vi "Pressure_control_subVI _newturbo.vi"(7 "Run Sequence":bool, 8 "user sequence, present (s) in, current step in, seq time in":T6, 9 "pressure parameters in":T3={"valve % open"=100.0, "Desired pressure"=0.0, "set Vapor sccm"=0.0, "set Gas sccm"=0.0, "Valve mode"=enum."% Open", "Pressure Mode"=enum."Abs. pressure", "analyte partial pressure"=100.0} caption="Set pressure parameters" {"analyte partial pressure" min=0.0 max=100.0 step=5.0; "set Gas sccm" min=0 max=200 step=5; "set Vapor sccm" min=0 max=200 step=5; "Desired pressure" min=0.0 max=760.0 step=5.0; "valve % open" min=0.0 max=100.0 step=5.0 format="%#_2f"}, 11 "pressure control on?/daq IDs/errors":T2) -> (0 "current step # out, shift register time out, seq button on?":T5, 1 "sequence over? USE THIS TO REINITIALIZE RUN SEQUENCE BUTTON SO PROGRAM ENDS":bool, 2 "save press/RH/gasflow/vaporflow - read valve position/pressure/vaporflow/gasflow":T4, 3 "pressure control on?/daq IDs/errors out":T1, 4 "sequence end date/time string":string, 5 "pressure_setpoint":string)   [LabVIEW 2014]
uses:
  <vilib>/DAQmx/read.llb/DAQmx Read (Analog 1D DBL NChan 1Samp).vi
  <vilib>/DAQmx/write.llb/DAQmx Write (Analog 1D DBL NChan 1Samp).vi
panel:
  # "100%"
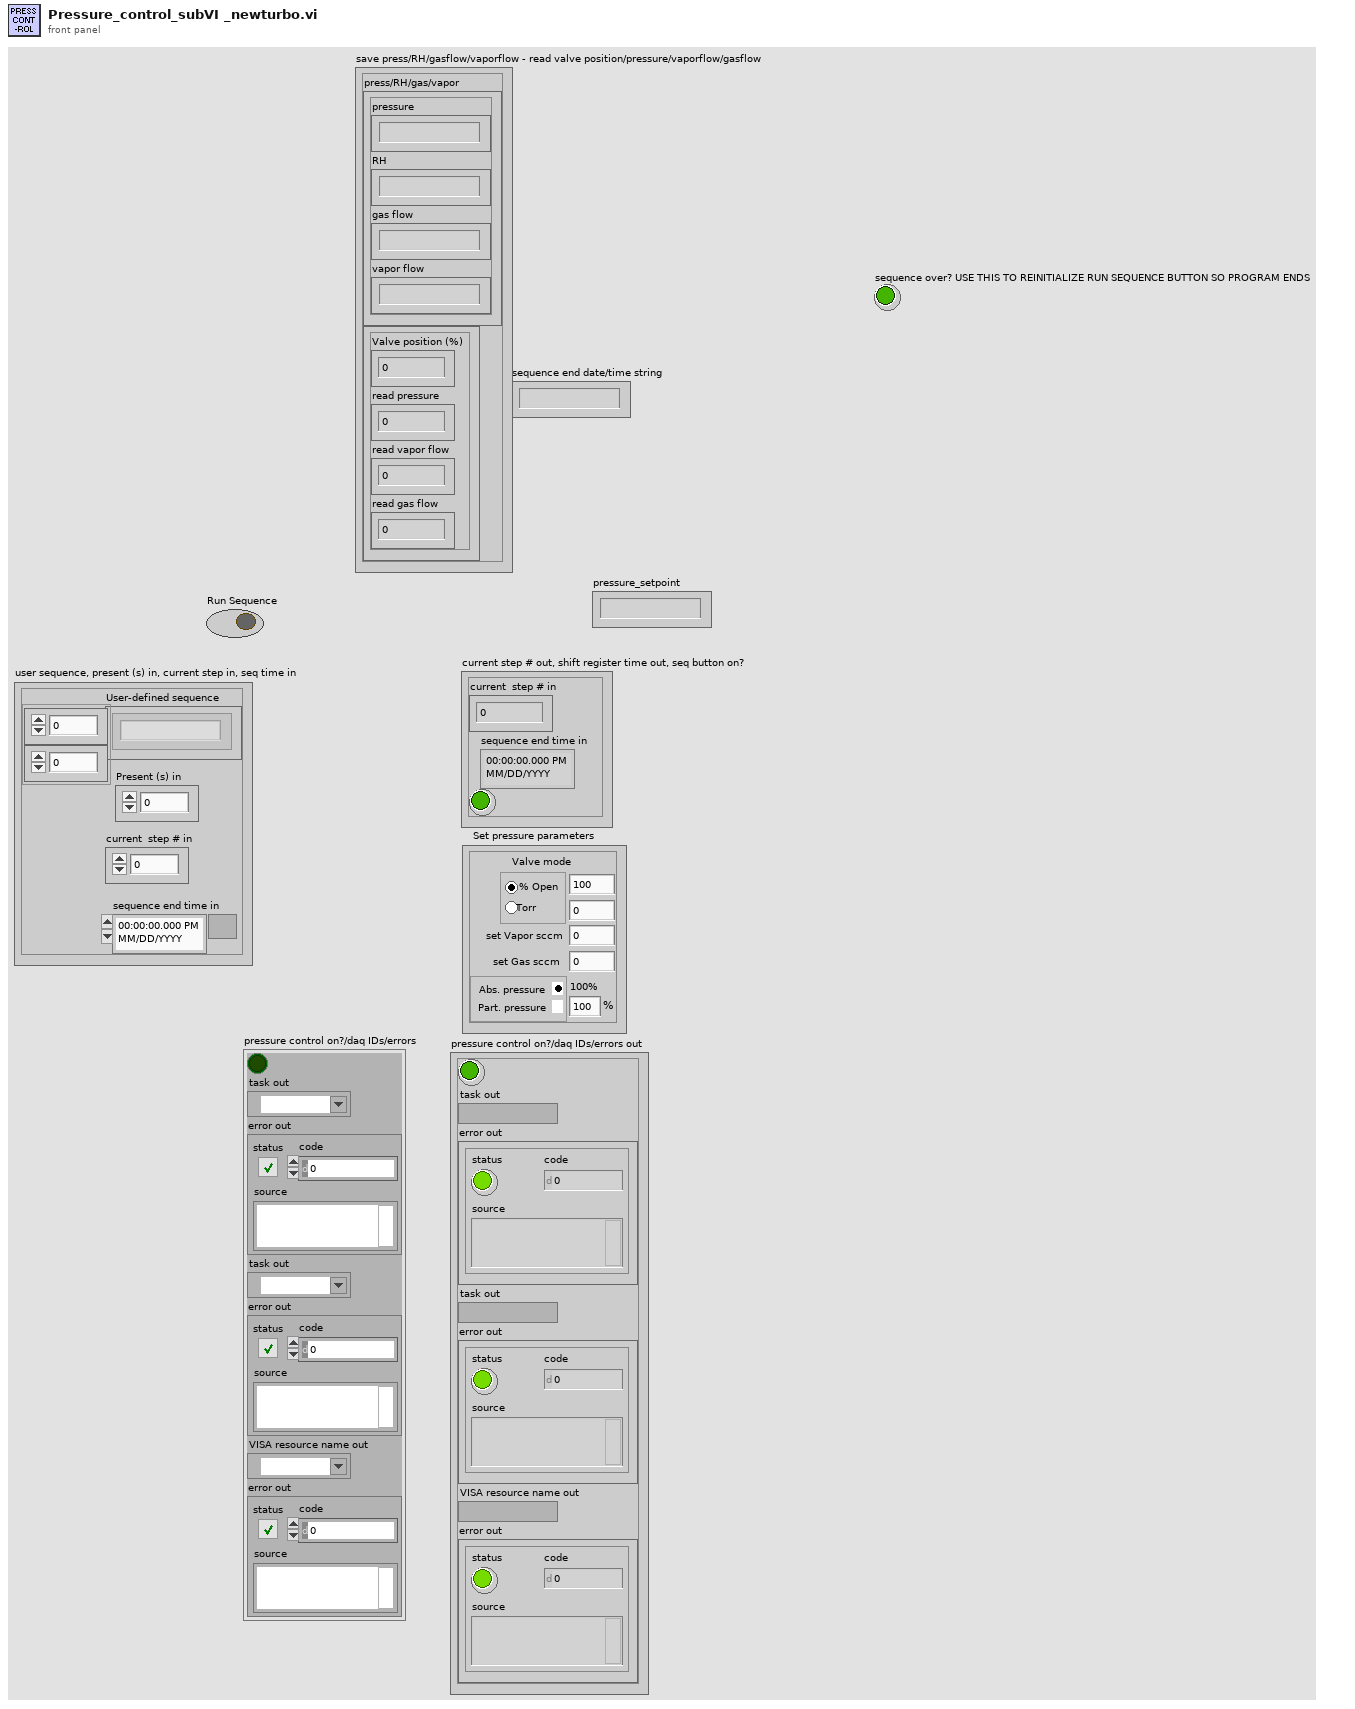
[diagram p1: front panel]
types:
  T1 = cluster{"Boolean":bool, "task out":refnum<k21>, "error out":errorcluster, "task out":refnum<k21>, "error out":errorcluster, "VISA resource name out":refnum<visa-resource-name>, "error out":errorcluster}
  T2 = cluster{bool, "task out":refnum<k21>, "error out":errorcluster, "task out":refnum<k21>, "error out":errorcluster, "VISA resource name out":refnum<visa-resource-name>, "error out":errorcluster}
  T3 = cluster{"valve % open":dbl, "Desired pressure":dbl, "set Vapor sccm":sgl, "set Gas sccm":sgl, "Valve mode":enum32{"% Open", "Torr "}, "Pressure Mode":enum32{"Abs. pressure", " Part. pressure"}, "analyte partial pressure":dbl}
  T4 = cluster{"press/RH/gas/vapor":cluster{"pressure":string, "RH":string, "gas flow":string, "vapor flow":string}, "Cluster":cluster{"Valve position (%)":dbl, "read pressure":dbl, "read vapor flow":dbl, "read gas flow":dbl}}
  T5 = cluster{"current  step # in":i32, "sequence end time in":timestamp, "Boolean":bool}
  T6 = cluster{"User-defined sequence":string[][], "Present (s) in":dbl, "current  step # in":i32, "sequence end time in":timestamp}
  T7 = cluster{"Valve position (%)":dbl, "pressure":dbl, "vapor flow":dbl, "gas flow":dbl}
  T8 = cluster{"pressure":string, "RH":string, "gas flow":string, "vapor flow":string}
  T9 = cluster{"String":dbl, "String":dbl, "Pressure Control":u32}
  T10 = cluster{"Valve position (%)":dbl, "read pressure":dbl, "read vapor flow":dbl, "read gas flow":dbl}
  T11 = cluster{bool, "task out":refnum<k21>, "error out":errorcluster, "task out":refnum<k21>, "error out":errorcluster, "VISA Refnum out":refnum<visa-resource-name>, "error out":errorcluster}
  T12 = cluster{"press/RH/gas/vapor":cluster{"pressure":string, "RH":string, "gas flow":string, "vapor flow":string}, cluster{"Valve position (%)":dbl, "read pressure":dbl, "read vapor flow":dbl, "read gas flow":dbl}}
  T13 = cluster{"current  step # in":i32, "sequence end time in":timestamp, bool}
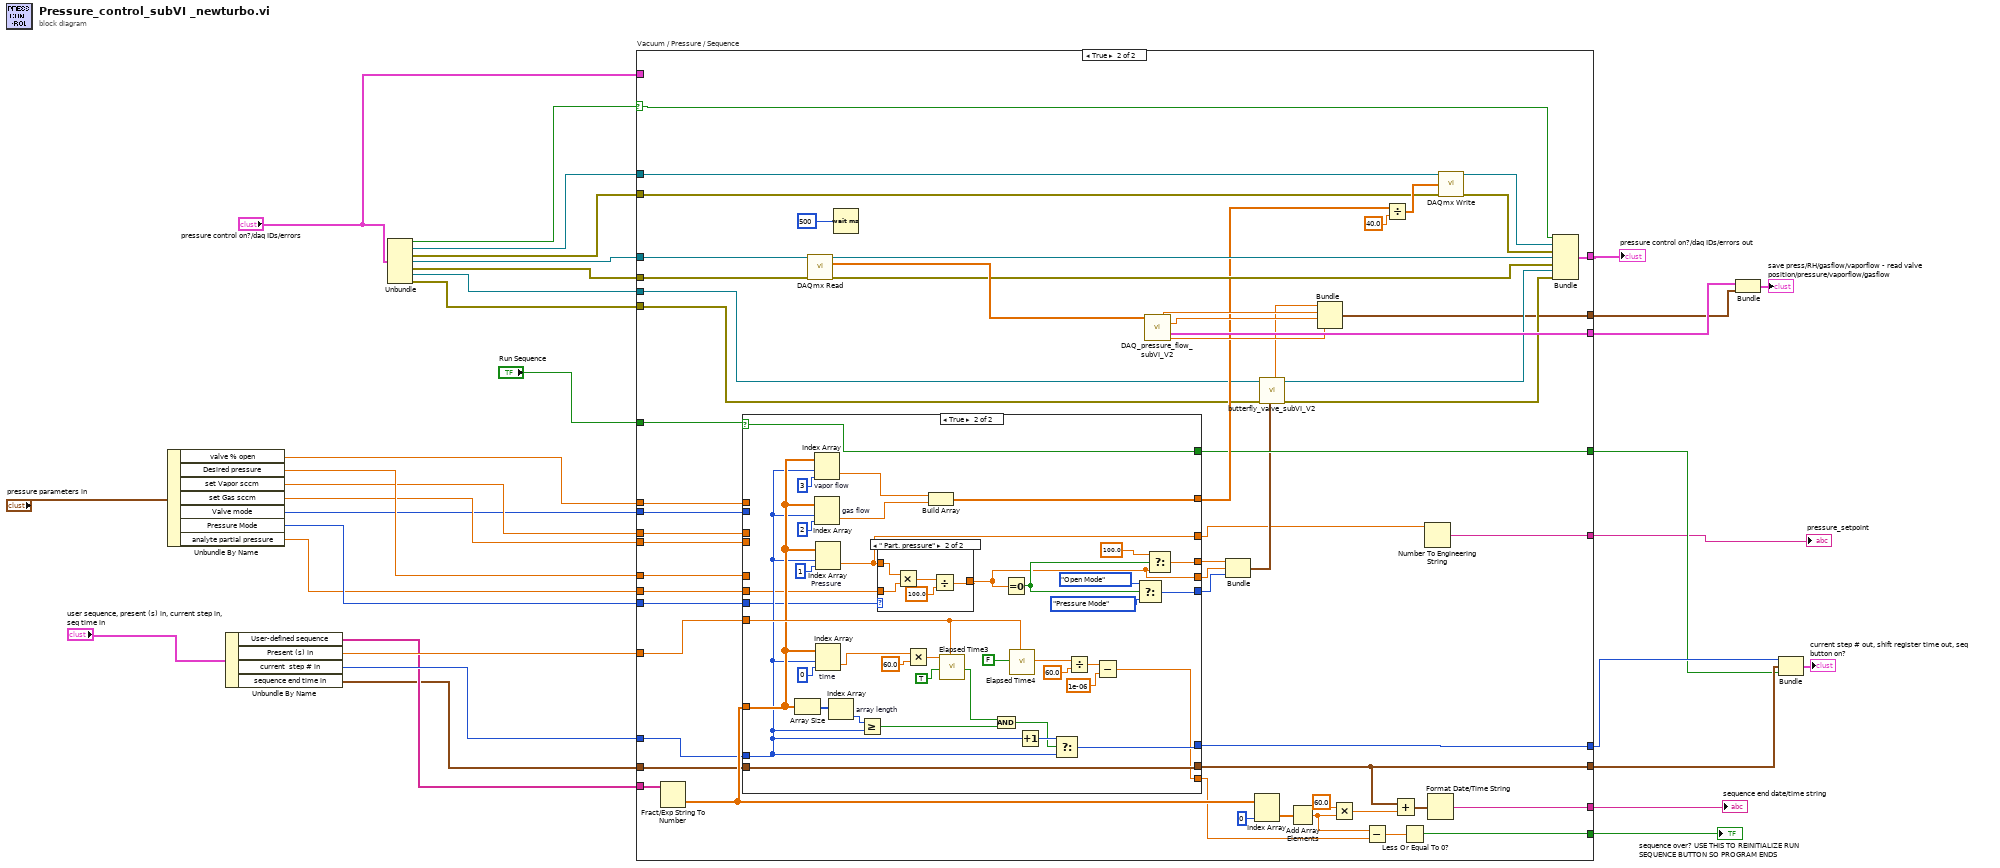
[diagram p0: block diagram]
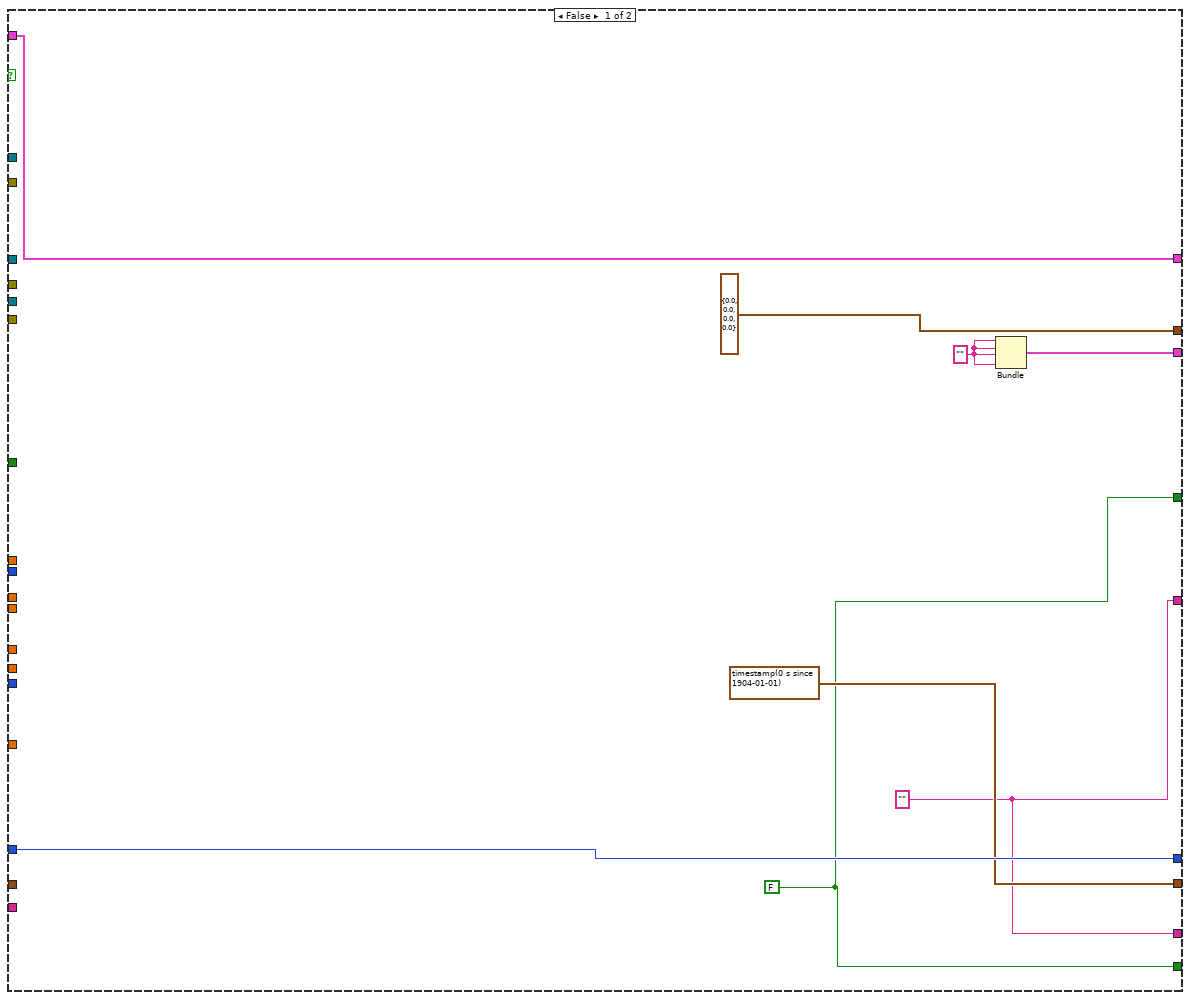
[diagram p2: hidden frame]
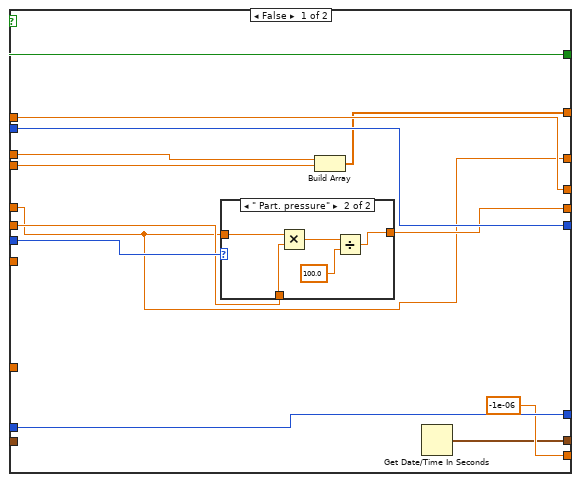
[diagram p3: hidden frame]
diagram:
  n1 = Unbundle By Name("pressure parameters in") -> ("valve % open"=w11:dbl, "Desired pressure"=w15:dbl, "set Vapor sccm"=w13:sgl, "set Gas sccm"=w14:sgl, "Valve mode"=w12:enum32{"% Open", "Torr "}, "Pressure Mode"=w17:enum32{"Abs. pressure", " Part. pressure"}, "analyte partial pressure"=w16:dbl)
  n2 = Unbundle By Name("user sequence, present (s) in, current step in, seq time in") -> ("User-defined sequence"=w27:string[][], "Present (s) in"=w28:dbl, "current  step # in"=w29:i32, "sequence end time in"=w26:timestamp)
  n3 = Unbundle("pressure control on?/daq IDs/errors") -> (w9:bool, "task out"=w8:refnum<k21>, "error out"=w7:errorcluster, "task out"=w6:refnum<k21>, "error out"=w5:errorcluster, "VISA resource name out"=w4:refnum<visa-resource-name>, "error out"=w3:errorcluster)
  n4 = case "Vacuum / Pressure / Sequence" shown="True" w9 {
    selector: w9 -> [_ w42]
    tunnel: w29 -> [w41 w73]
    tunnel: [w41 w53] -> w25
    tunnel: [w36 w71] -> w23
    tunnel: [timestamp(0 s since 1904-01-01) ("seconds since 1Jan1904") w70] -> w24
    tunnel: [w39 w87] -> w21
    tunnel: w27 -> [_ w78]
    tunnel: [w35 w77] -> w33
    tunnel: [T7 {"Valve position (%)"=0.0, "pressure"=0.0, "vapor flow"=0.0, "gas flow"=0.0} w76] -> w20
    tunnel: w28 -> [_ w68]
    tunnel: "Run Sequence" -> [_ w67]
    tunnel: w26 -> [_ w66]
    tunnel: [w36 w65] -> w31
    tunnel: w15 -> [_ w64]
    tunnel: w11 -> [_ w63]
    tunnel: w13 -> [_ w62]
    tunnel: w17 -> [_ w61]
    tunnel: w12 -> [_ w60]
    tunnel: w14 -> [_ w59]
    tunnel: w16 -> [_ w58]
    tunnel: [w35 w50] -> w10
    tunnel: w8 -> [_ w49]
    tunnel: w7 -> [_ w48]
    tunnel: w6 -> [_ w47]
    tunnel: w5 -> [_ w46]
    tunnel: w4 -> [_ w45]
    tunnel: w3 -> [_ w44]
    tunnel: "pressure control on?/daq IDs/errors" -> [w34 _]
    tunnel: [w34 w43] -> w1
    frame False {
      w35 = "" ("date/time string")
      w36 = FALSE
      w38 = ""
      n5 = Bundle(w38, w38, w38, w38) -> (w39:cluster{string, string, string, string})  [unwired: 1 in]
    }
    frame True {
      n6 = Fract/Exp String To Number ("user sequence")(string=w78) -> (number=w74:dbl[][])  [unwired: 3 in, 1 out]
      n7 = case "Sequence" shown="True" w67 {
        selector: w67 -> [w108 w137]
        tunnel: w68 -> [_ w145]
        tunnel: [w111 w146] -> w53
        tunnel: w73 -> [w111 w138]
        tunnel: w59 -> [w106 _]
        tunnel: [w103 w118] -> w57
        tunnel: w74 -> [_ w140]
        tunnel: w60 -> [w110 _]
        tunnel: [w110 w123] -> w56
        tunnel: [-1e-06 w120] -> w69
        tunnel: [w108 w137] -> w71
        tunnel: [w107 w127] -> w52
        tunnel: w63 -> [w107 _]
        tunnel: [w105 w133] -> w72
        tunnel: [w104 w132] -> w70
        tunnel: w66 -> [_ w132]
        tunnel: w64 -> [w99 _]
        tunnel: w58 -> [w100 w131]
        tunnel: w61 -> [w102 w129]
        tunnel: w62 -> [w101 _]
        tunnel: [w99 w119] -> w51
        frame False {
          n8 = case shown="\" Part. pressure\"" w102 {
            tunnel: [w112 w113] -> w103
            tunnel: w99 -> [w112 w115]
            tunnel: w100 -> [_ w114]
            frame "Abs. pressure", Default {
            }
            frame " Part. pressure" {
              n9 = Multiply(x=w115, y=w114) -> (x*y=w117:dbl)
              n10 = Divide(x=w117, y=100.0 ("Analyte part. press. (%)")) -> (x/y=w113:dbl)
            }
          }
          n11 = Build Array(w101, w106) -> (w105:sgl[])
          n12 = Get Date/Time In Seconds() -> (seconds since 1Jan1904=w104:timestamp)
        }
        frame True {
          n13 = Array Size(array=w140) -> (size(s)=w156:i32[])
          n14 = Index Array "vapor flow"(array=w140, index (row)=w138, index (col)=3 ("disabled index (col)")) -> (element=w135:dbl)
          n15 = Index Array "gas flow"(array=w140, index (row)=w138, index (col)=2 ("disabled index (col)")) -> (element=w134:dbl)
          n16 = Index Array "Pressure"(array=w140, index (row)=w138, index (col)=1 ("disabled index (col)")) -> (element=w119:dbl)
          n17 = Index Array "time"(array=w140, index (row)=w138, index (col)=0) -> (element=w149:dbl)
          n18 = Index Array "array length"(array=w156) -> (element=w141:i32)  [unwired: 1 in]
          n19 = Greater Or Equal?(x=w141, y=w138) -> (x >= y?=w153:bool)
          n20 = case shown="\" Part. pressure\"" w129 {
            tunnel: [w157 w158] -> w118
            tunnel: w119 -> [w157 w160]
            tunnel: w131 -> [_ w159]
            frame "Abs. pressure", Default {
            }
            frame " Part. pressure" {
              n21 = Multiply(x=w160, y=w159) -> (x*y=w161:dbl)
              n22 = Divide(x=w161, y=100.0 ("Analyte part. press. (%)")) -> (x/y=w158:dbl)
            }
          }
          n23 = Multiply(x=w149, y=60.0) -> (x*y=w139:dbl)
          n24 = Build Array(w135, w134) -> (w133:dbl[])
          n25 = call "Elapsed Time3"("Time Target (s)"=w139, "Auto Reset"=TRUE, "Set Start Time (s)"=w145) -> ("Time has Elapsed"=w130:bool)  [unwired: 9 in, 7 out]
          n26 = And(x=w130, y=w153) -> (x .and. y?=w136:bool)
          n27 = Equal To 0?(x=w118) -> (x = 0?=w126:bool)
          n28 = call "Elapsed Time4"("Reset"=FALSE, "Set Start Time (s)"=w145) -> ("Elapsed Time (s)"=w143:dbl)  [unwired: 10 in, 7 out]
          n29 = Increment(x=w138) -> (x+1=w147:i32)
          n30 = Select(t=w147, s=w136, f=w138) -> (s? t:f=w146:i32)
          n31 = Divide(x=w143, y=60.0) -> (x/y=w122:dbl)
          n32 = Subtract(x=w122, y=1e-06) -> (x-y=w120:dbl)
          n33 = Select(t=enum32{"Open Mode", "Pressure Mode"}."Open Mode" ("Pressure Control"), s=w126, f=enum32{"Open Mode", "Pressure Mode"}."Pressure Mode" ("Pressure Control")) -> (s? t:f=w123:enum32{"Open Mode", "Pressure Mode"})
          n34 = Select(t=100.0 ("valve % open 2"), s=w126, f=w118) -> (s? t:f=w127:dbl)
        }
      }
      n35 = call-poly <vilib>:"DAQmx Read.vi"("task/channels in"=w47, "error in"=w46) -> ("task out"=w84:refnum<k21>, "data"=w97:dbl[], "error out"=w83:errorcluster)  [unwired: 11 in]
      n36 = Wait (ms)(milliseconds to wait=u32 500) -> ()  [unwired: 1 out]
      n37 = call "DAQ_pressure_flow_subVI_V2.vi"("vac press"=w97) -> ("read pressure"=w75:dbl, "read vapor flow"=w80:dbl, "press/RH/gas/vapor"=w87:T8, "read gas flow"=w79:dbl)  [unwired: 11 in]
      n38 = Bundle("String"=w52, "String"=w57, "Pressure Control"=w56) -> (w54:T9)  [unwired: 1 in]
      n39 = Index Array(array=w74, index (col)=0 ("disabled index (col)")) -> (element=w94:dbl[])  [unwired: 1 in]
      n40 = call "butterfly_valve_subVI_V2.vi"("% open / desired pressure / pressure mode"=w54, "error in (no error)"=w44, "VISA Refnum in"=w45) -> ("error out"=w81:errorcluster, "VISA Refnum out"=w82:refnum<visa-resource-name>, "Valve position (%)"=w55:dbl)  [unwired: 6 in]
      n41 = Add Array Elements(numeric array=w94) -> (sum=w88:dbl)
      n42 = Bundle("Valve position (%)"=w55, "read pressure"=w75, "read vapor flow"=w80, "read gas flow"=w79) -> (w76:T10)  [unwired: 1 in]
      n43 = Multiply(x=60.0 ("y"), y=w88) -> (x*y=w90:dbl)
      n44 = Subtract(x=w88, y=w69) -> (x-y=w92:dbl)
      n45 = Divide(x=w72, y=40.0 ("Waveform")) -> (x/y=w96:dbl[])
      n46 = Add(x=w70, y=w90) -> (x+y=w89:timestamp)
      n47 = Less Or Equal To 0?(x=w92) -> (x <= 0?=w65:bool)
      n48 = Number To Engineering String(4:w51) -> (0:w50:string)  [unwired: 3 in]
      n49 = Format Date/Time String(seconds (now)=w89) -> (date/time string=w77:string)  [unwired: 2 in]
      n50 = call-poly <vilib>:"DAQmx Write.vi"("task/channels in"=w49, "data"=w96, "error in"=w48) -> ("task out"=w86:refnum<k21>, "error out"=w85:errorcluster)  [unwired: 10 in, 1 out]
      n51 = Bundle(w42, "task out"=w86, "error out"=w85, "task out"=w84, "error out"=w83, "VISA Refnum out"=w82, "error out"=w81) -> (w43:T11)  [unwired: 1 in]
    }
  }
  "sequence end date/time string" <- w33
  "sequence over? USE THIS TO REINITIALIZE RUN SEQUENCE BUTTON SO PROGRAM ENDS" <- w31
  "pressure_setpoint" <- w10
  "pressure control on?/daq IDs/errors out" <- w1
  n52 = Bundle("press/RH/gas/vapor"=w21, w20) -> (→"save press/RH/gasflow/vaporflow - read valve position/pressure/vaporflow/gasflow":T12)  [unwired: 1 in]
  n53 = Bundle("current  step # in"=w25, "sequence end time in"=w24, w23) -> (→"current step # out, shift register time out, seq button on?":T13)  [unwired: 1 in]
